vi "Populate Scope.vi"(8 "Error In":errorcluster, 11 "State In":T1) -> (0 "Error Out":errorcluster, 3 "State Out":T1)   [LabVIEW 2017, in "Bookmark Manager.lvlib"]
uses:
  Bookmark Manager.lvlib
  Controls/State.ctl
  Controls/VI Bookmark.ctl
  Controls/VI Information.ctl
  Controls/Application Information.ctl
  Controls/Bookmarks Views.ctl
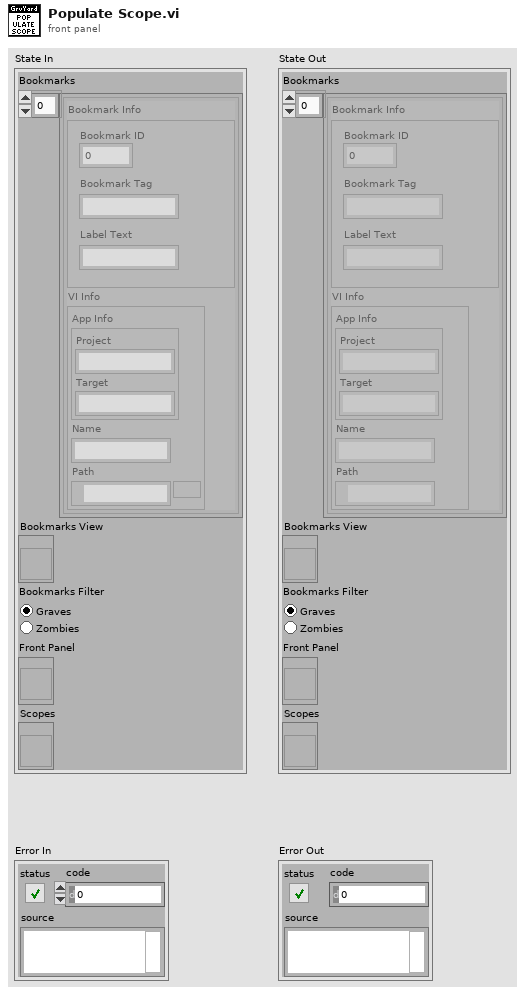
[diagram p1: front panel]
types:
  T1 = typedef "Bookmark Manager.lvlib/State.ctl" = cluster{"Bookmarks":T2[], "Bookmarks View":refnum<vi>, "Bookmarks Filter":T5, "Front Panel":refnum<vi>, "Scopes":refnum<vi>}
  T2 = typedef "Bookmark Manager.lvlib/VI Bookmark.ctl" = cluster{"Bookmark Info":cluster{"Bookmark ID":u32, "Bookmark Tag":string, "Label Text":string}, "VI Info":T3}
  T3 = typedef "Bookmark Manager.lvlib/VI Information.ctl" = cluster{"App Info":T4, "Name":string, "Path":path}
  T4 = typedef "Bookmark Manager.lvlib/Application Information.ctl" = cluster{"Project":string, "Target":string}
  T5 = typedef "Bookmark Manager.lvlib/Bookmarks Views.ctl" = enum32{"Graves", "Zombies"}
  T6 = enum8{"Enabled", "Disabled", "Disabled and Grayed Out"}
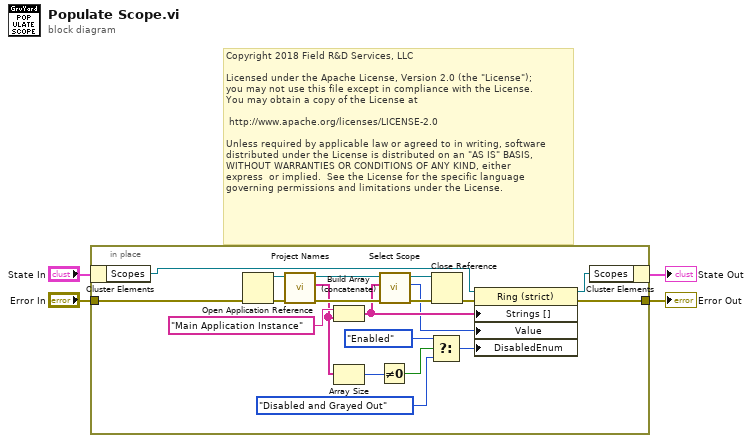
[diagram p0: block diagram]
diagram:
  # "Copyright 2018 Field R&D Services, LLC\n\nLicensed under the Apache License, Version 2.0 (the \"License\");\nyou may not use this file except in compliance with the License.\nYou may obtain a copy of the License at\n\n\thttp://www.apache.org/licenses/LICENSE-2.0\n\nUnless required by applicable law or agreed to in writing, software\ndistributed under the License is distributed on an \"AS IS\" BASIS,\nWITHOUT WARRANTIES OR CONDITIONS OF ANY KIND, either \nexpress  or implied.  See the License for the specific language \ngoverning permissions and limitations under the License."
  n1 = in-place {
    in-place-border: "Error In" -> [w22]
    in-place-border: [w23] -> w3
    n2 = in-place-cluster #1("State In") -> ("Scopes"=w7:refnum<vi>)
    n3 = Open Application Reference(8:w22) -> (0:w21:errorcluster, 3:w20:refnum<vi>)  [unwired: 3 in]
    n4 = call "Project Names.vi"("Error In"=w21, "App In"=w20) -> ("Error Out"=w18:errorcluster, "Project Names"=w10:string[], "App Out"=w19:refnum<vi>)  [unwired: 7 in]
    n5 = Build Array (concatenate)("Main Application Instance", w10) -> (w6:string[])
    n6 = Array Size(array=w10) -> (size(s)=w9:i32)
    n7 = Not Equal To 0?(x=w9) -> (x != 0?=w8:bool)
    n8 = call "Select Scope.vi"("Error In"=w18, "Strings[]"=w6, "App In"=w19) -> ("Error Out"=w15:errorcluster, "Selection"=w5:u16, "App Out"=w16:refnum<vi>)  [unwired: 6 in]
    n9 = Select(t=T6."Enabled" ("Disabled"), s=w8, f=T6."Disabled and Grayed Out" ("Disabled")) -> (s? t:f=w12:T6)
    n10 = Close Reference(reference=w16, error in (no error)=w15) -> (error out=w17:errorcluster)
    n11 = property class="Ring (strict)"(reference=w7, error in=w17, "Strings []"=w6, "Value"=w5, "DisabledEnum"=w12) -> (reference out=w24:refnum<vi>, error out=w23:errorcluster)
    n12 = in-place-cluster #1("Scopes"=w24) -> (→"State Out":T1)
  }
  "Error Out" <- w3
